vi "FPGA_PPG_query_error.vi"(0 "resource_in":refnum<visa-resource-name>, 5 "error in (no error)":errorcluster) -> (14 "resource_out":refnum<visa-resource-name>, 19 "error out":errorcluster)   [LabVIEW 2014, in "NI-FPGA_PPG_Driver.lvlib"]
doc: "Queries the last error of the FPGA.\n\nContact: Falk Ziegler, eMail: ziegler@physik.uni-greifswald.de"
uses:
  NI-FPGA_PPG_Driver.lvlib
  <vilib>/rvi/interface/nirviReadWriteControl/nirviReadWriteControl.xnode
  FPGA_PPG_action_type.ctl
  FPGA_PPG_vi_ref.ctl
  FPGA Bitfiles/TiTaProj_COF_PPG_100MHz.lvbitx
  <vilib>/rvi/errors/niLvFpgaMergeErrorWithErrorCode.vi
  <vilib>/rvi/errors/niLvFpgaAdjustHostInterfaceError.vi
  FPGA_PPG_error_type.ctl
panel:
  in  "errorCodes":T1
  out "errorMessage":string
  out "errorCode":i32[](array[numeric])
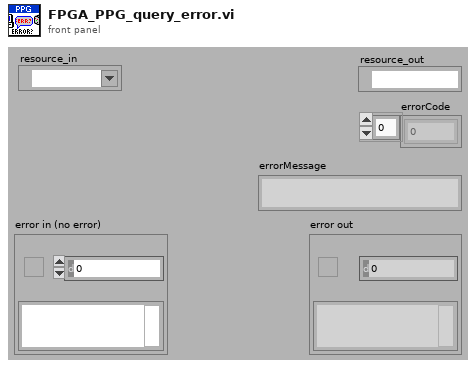
[diagram p1: front panel]
types:
  T1 = typedef "NI-FPGA_PPG_Driver.lvlib/FPGA_PPG_error_type.ctl" = enum16{"no error", "resource not initialized (no commands and invalid mem address)", "wrong memory address (address > Nof commands)", "invalid time value (probably too short)", "cannot start FPGA because one or more errors occured", "FIFO (internal) empty unexpectedly", "DMA FIFO (download from host) full unexpectedly", "checking number of commands: failed", "unknown error 8", "unknown error 9", "unknown error 10", "unknown error 11", "unknown error 12", "unknown error 13", "unknown error 14", "unknown error 15", "unknown error 16", "unknown error 17", "unknown error 18", "unknown error 19", "can't change state while pattern output is in progress"}
  T2 = typedef "NI-FPGA_PPG_Driver.lvlib/FPGA_PPG_action_type.ctl" = enum16{"GET", "SET", "REMOVE"}
  T3 = typedef "NI-FPGA_PPG_Driver.lvlib/FPGA_PPG_vi_ref.ctl" = refnum<k20>
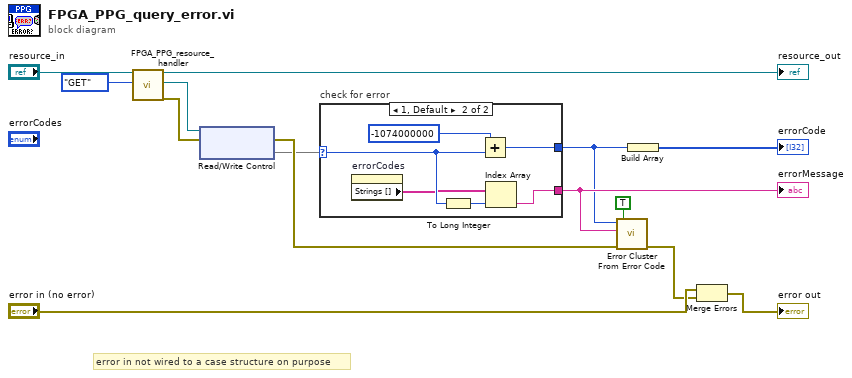
[diagram p0: block diagram]
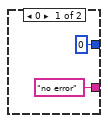
[diagram p2: hidden frame]
diagram:
  # "error in not wired to a case structure on purpose"
  n1 = call "FPGA_PPG_resource_handler.vi"("resource_in"="resource_in", "action"=FPGA_PPG_action_type."GET") -> ("resource_out"=→"resource_out":refnum<visa-resource-name>, "FPGA VI Reference Out"=w1:T3, "error out"=w13:errorcluster)  [unwired: 15 in]
  n2 = xnode "Read/Write Control"("FPGA VI Reference In"=w1, "error in"=w13) -> ("error out"=w6:errorcluster, "error_code"=w5)  [unwired: 1 out]
  n3 = case "check for error" shown="1, Default" w5 {
    selector: w5 -> [_ w20]
    tunnel: [0 w21] -> w3
    tunnel: ["no error" w19] -> w4
    frame 0 {
    }
    frame 1, Default {
      n4 = property on="errorCodes" class="Enum (strict)"() -> ("Strings []"=w18:string[])  [unwired: 2 in, 2 out]
      n5 = To Long Integer(number=w20) -> (32bit integer=w17:i32)
      n6 = Add(x=-1074000000 ("error code (0)"), y=w20) -> (x+y=w21:i32)
      n7 = Index Array(array=w18, index=w17) -> (element=w19:string)
    }
  }
  "errorMessage" <- w4
  n8 = call <vilib>:"Error Cluster From Error Code.vi"("show call chain? (False)"=TRUE, "error in (no error)"=w6, "error message (\"\")"=w4, "error code (0)"=w3) -> ("error out"=w11:errorcluster)  [unwired: 5 in]
  n9 = Build Array(w3) -> (→"errorCode":i32[])
  n10 = Merge Errors("error in (no error)", w11) -> (→"error out":errorcluster)
